vi "Last char received.vi"(10 "Receive string":string, 11 "Command":string="$") -> (3 "Command Received":bool)   [LabVIEW 2015]
panel:
  out "index of element":i32
  out "element":u8
  out "unsigned byte array":u8[](array[numeric])
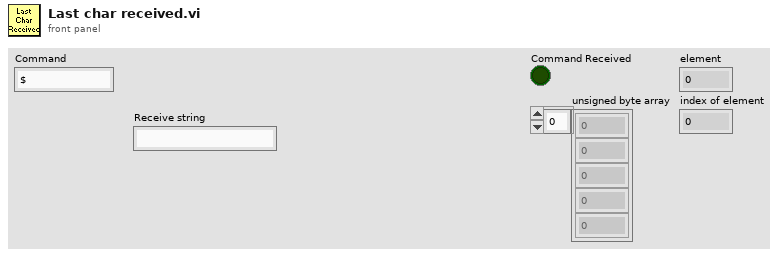
[diagram p1: front panel]
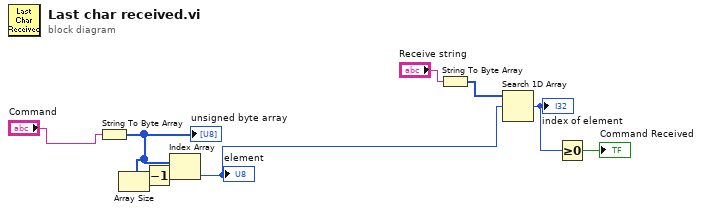
[diagram p0: block diagram]
diagram:
  n1 = String To Byte Array(string="Command") -> (unsigned byte array=w9:u8[])
  "unsigned byte array" <- w9
  n2 = Array Size(array=w9) -> (size(s)=w8:i32)
  n3 = Decrement(x=w8) -> (x-1=w7:i32)
  n4 = Index Array(array=w9, index=w7) -> (element=w4:u8)
  "element" <- w4
  n5 = String To Byte Array(string="Receive string") -> (unsigned byte array=w5:u8[])
  n6 = Search 1D Array(1D array=w5, element=w4) -> (index of element=w2:i32)  [unwired: 1 in]
  "index of element" <- w2
  n7 = Greater Or Equal To 0?(x=w2) -> (x >= 0?=→"Command Received":bool)
